vi "Check Sum Test_01.vi"(10 "Array":string[](array[string]), 11 "ToolString Input":string="$AGENT,53,VS-62U009+VS-69W014*71") -> (1 "ToolStringOut_01":string, 2 "ChkSum":string, 3 "x = y?":bool)   [LabVIEW 2019]
panel:
  out "ChkSum2":string
  out "ChkSum1":string
  out "ASCII 格式輸出 2":string
  out "ASCII 格式輸出":string
  out "number 3":u32
  out "number 2":u32
  out "Rad In Reg 2":string
  out "hex integer string":string[](array[string])
  out "unsigned byte array":u8[](array[numeric]) format="%x"
  out "Rad In Reg":string
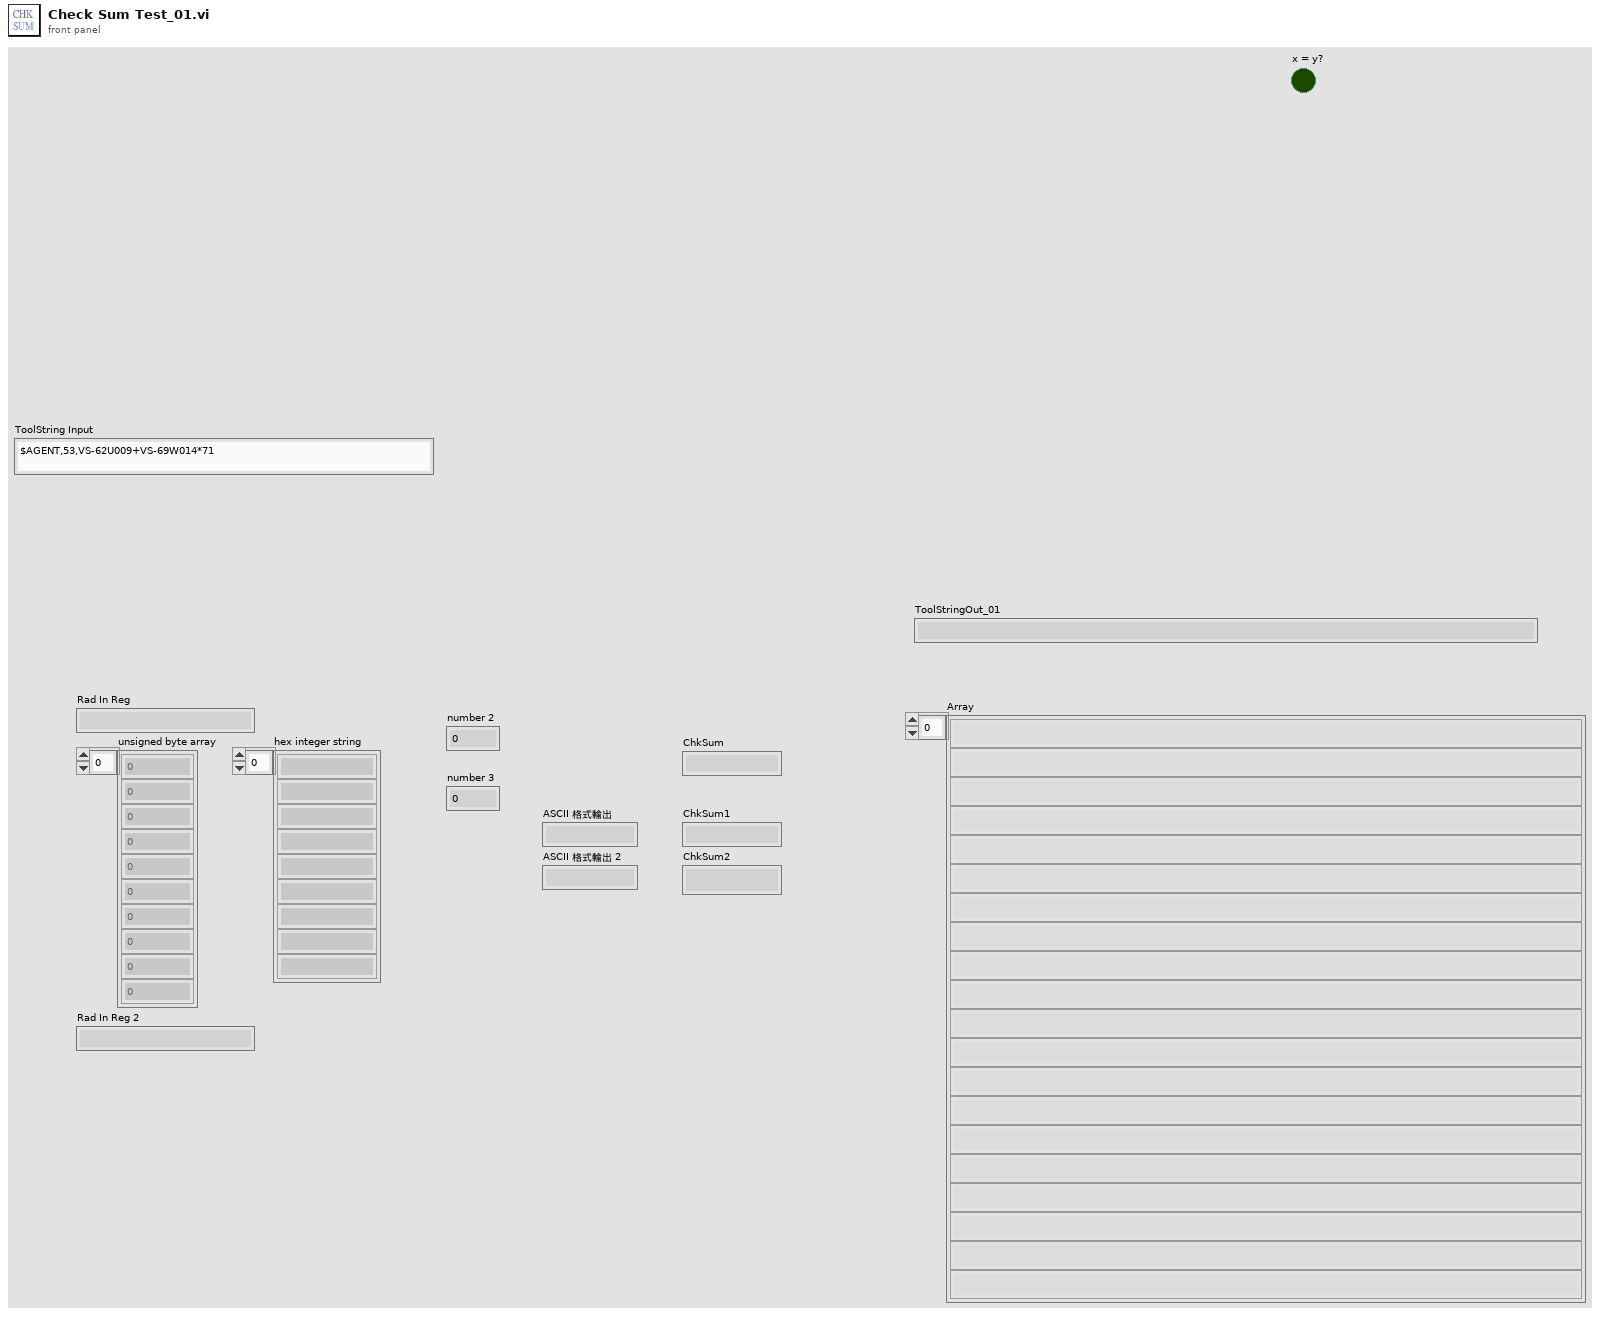
[diagram p1: front panel]
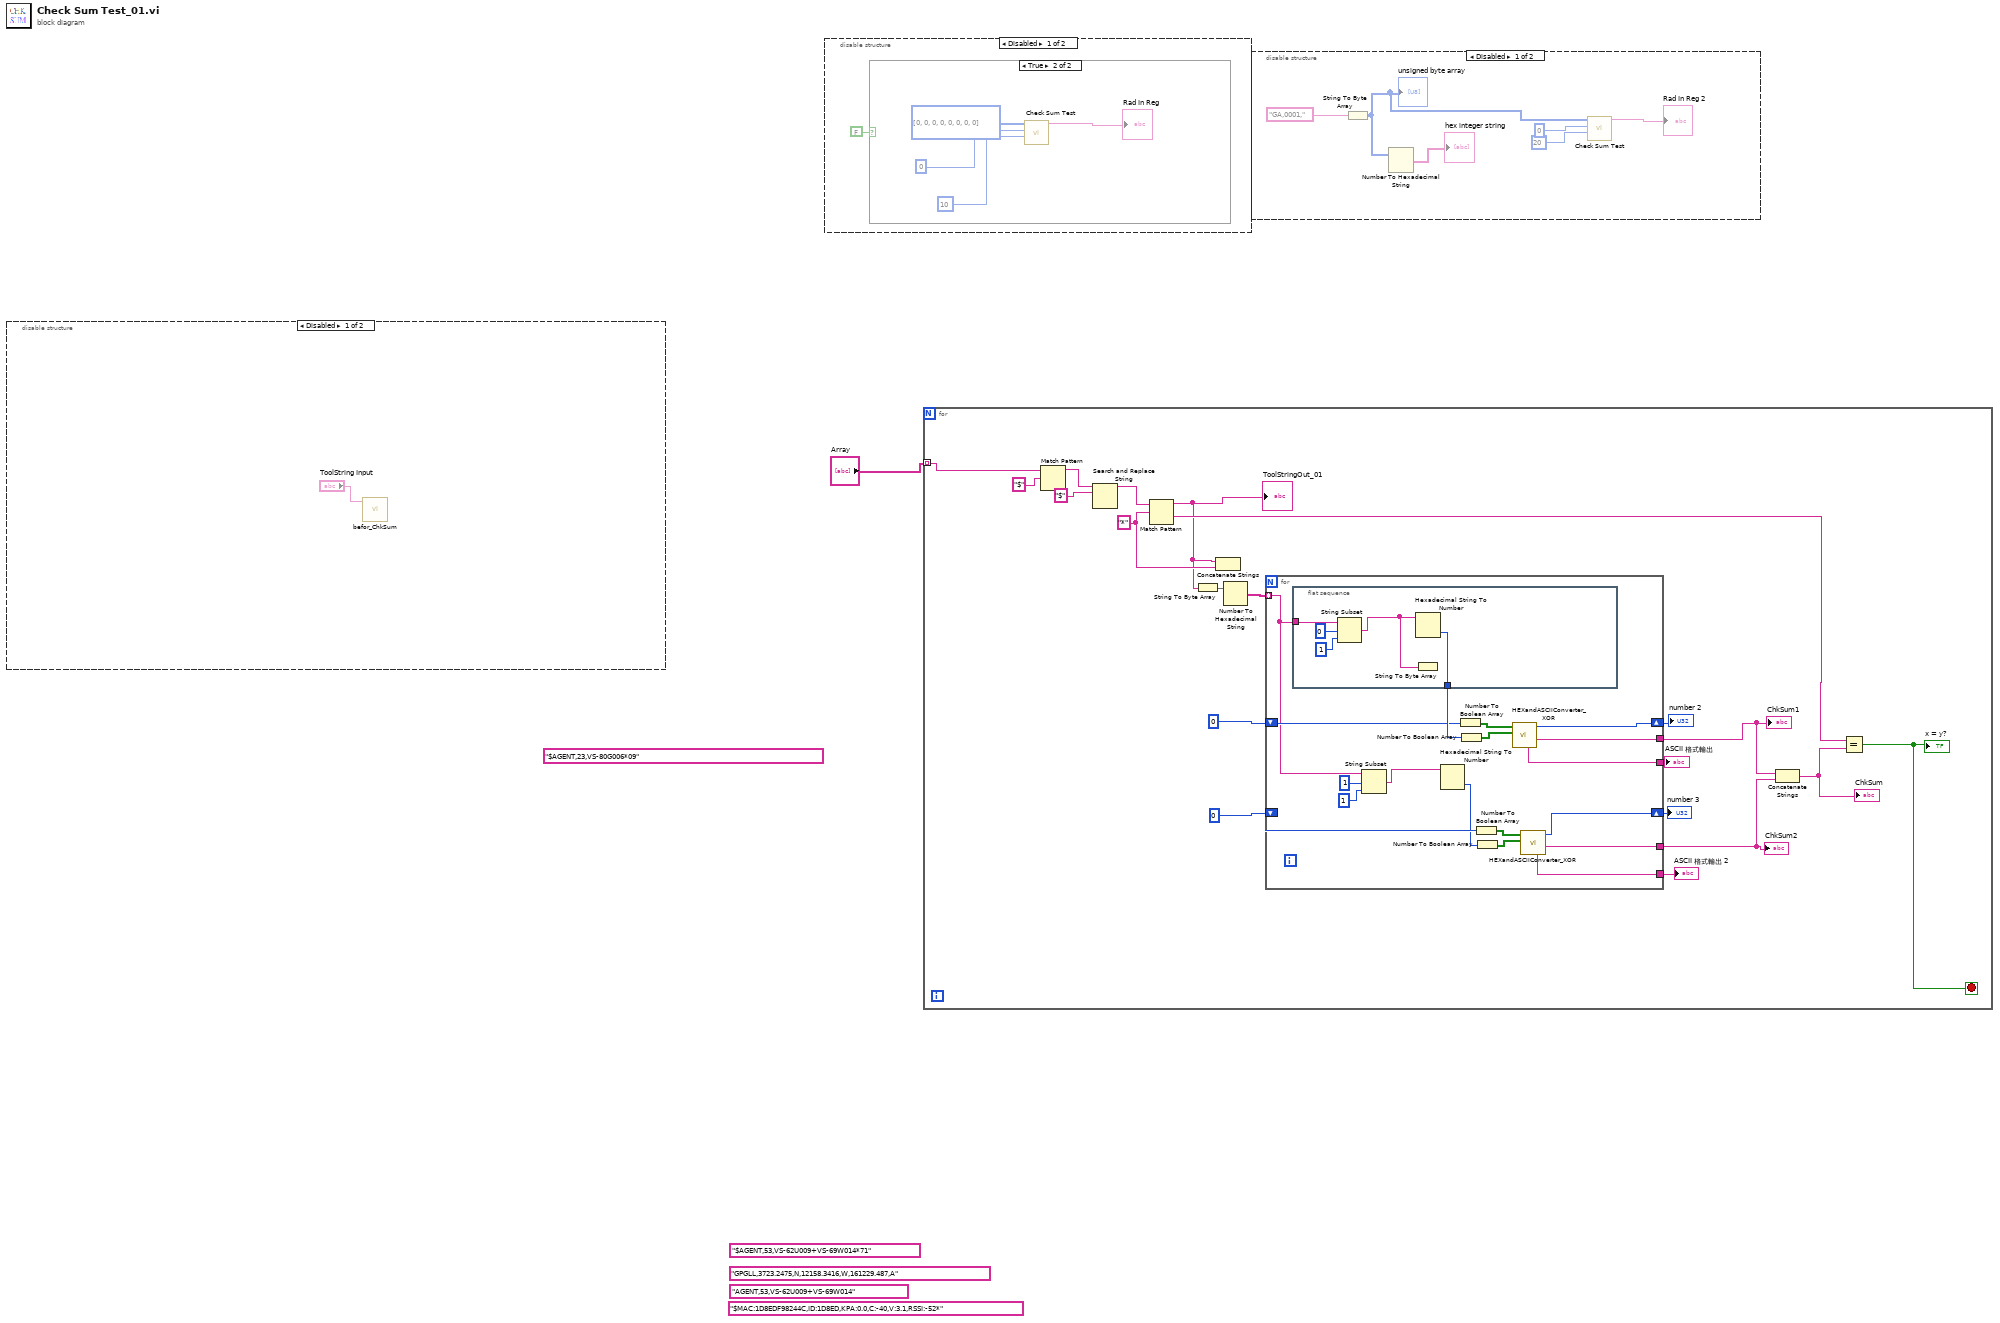
[diagram p0: block diagram]
diagram:
  (unwired) "$AGENT,23,VS-80G006*09"
  (unwired) "$AGENT,53,VS-62U009+VS-69W014*71"
  (unwired) "$MAC:1D8EDF98244C,ID:1D8ED,KPA:0.0,C:-40,V:3.1,RSSI:-52*"
  (unwired) "GPGLL,3723.2475,N,12158.3416,W,161229.487,A"
  (unwired) "AGENT,53,VS-62U009+VS-69W014"
  n1 = disable-structure shown="Disabled" {
    frame Disabled {
      n2 = call "befor_ChkSum.vi"("ToolString Input"="ToolString Input") -> ()  [unwired: 10 in, 1 out]
    }
    frame Enabled {
    }
  }
  n3 = disable-structure shown="Disabled" {
    frame Disabled {
      n4 = case shown="True" FALSE {
        frame False {
        }
        frame True {
          n5 = call "Check Sum Test.vi"("length"=10, "index"=0, "Input Registers Arr"=u16[] [0, 0, 0, 0, 0, 0, 0, 0]) -> ("Rad In Reg"=→"Rad In Reg":string)  [unwired: 8 in]
        }
      }
    }
    frame Enabled {
    }
  }
  n6 = for {
    tunnel: "Array" -> [w10] mode=indexing
    stop <- w9 stop-if-true
    w15 = "*" ("regular expression")
    n7 = Match Pattern(string=w10, regular expression="$") -> (before substring=w17:string)  [unwired: 1 in, 3 out]
    n8 = Search and Replace String(input string=w17, search string="$" ("regular expression")) -> (result string=w16:string)  [unwired: 6 in, 3 out]
    n9 = Match Pattern(string=w16, regular expression=w15) -> (before substring=w8:string, after substring=w12:string)  [unwired: 1 in, 2 out]
    "ToolStringOut_01" <- w8
    n10 = String To Byte Array(string=w8) -> (unsigned byte array=w23:u8[])
    n11 = Concatenate Strings(w8, w15) -> ()  [unwired: 1 out]
    n12 = Number To Hexadecimal String(2:w23) -> (0:w20:string[])  [unwired: 1 in]
    n13 = for {
      tunnel: w20 -> [w37] mode=indexing
      shift-right: [w41] -> w26
      shift-left: 0 -> [w42]
      shift-right: [w32] -> w24
      shift-left: 0 -> [w34]
      tunnel: [w31] -> w22
      tunnel: [w30] -> w21
      tunnel: [w29] -> w14
      tunnel: [w28] -> w13
      n14 = flat-sequence {
        tunnel: w37 -> [w48]
        tunnel: [w46] -> w43
        frame #0 {
          n15 = String Subset(string=w48, offset (0)=0, length (rest)=1) -> (substring=w47:string)
          n16 = Hexadecimal String To Number(string=w47) -> (number=w46:u32)  [unwired: 2 in, 1 out]
          n17 = String To Byte Array(string=w47) -> ()  [unwired: 1 out]
        }
      }
      n18 = String Subset(string=w37, offset (0)=1, length (rest)=1) -> (substring=w40:string)
      n19 = Hexadecimal String To Number(string=w40) -> (number=w33:u32)  [unwired: 2 in, 1 out]
      n20 = Number To Boolean Array(number=w42) -> (Boolean array=w45:bool[])
      n21 = Number To Boolean Array(number=w43) -> (Boolean array=w44:bool[])
      n22 = Number To Boolean Array(number=w34) -> (Boolean array=w35:bool[])
      n23 = Number To Boolean Array(number=w33) -> (Boolean array=w36:bool[])
      n24 = call "HEXandASCIIConverter_XOR.vi"("Boolean array2 in"=w44, "Boolean array1 in"=w45) -> ("hex integer string"=w29:string, "number"=w41:u32, "ASCII 格式輸出"=w31:string)  [unwired: 6 in, 1 out]
      n25 = call "HEXandASCIIConverter_XOR.vi"("Boolean array2 in"=w36, "Boolean array1 in"=w35) -> ("hex integer string"=w28:string, "number"=w32:u32, "ASCII 格式輸出"=w30:string)  [unwired: 6 in, 1 out]
    }
    "number 2" <- w26
    "number 3" <- w24
    "ASCII 格式輸出" <- w22
    "ASCII 格式輸出 2" <- w21
    "ChkSum1" <- w14
    "ChkSum2" <- w13
    n26 = Concatenate Strings(w14, w13) -> (w11:string)
    "ChkSum" <- w11
    n27 = Equal?(x=w12, y=w11) -> (x = y?=w9:bool)
    "x = y?" <- w9
  }
  n28 = disable-structure shown="Disabled" {
    frame Disabled {
      n29 = String To Byte Array(string="GA,0001,") -> (unsigned byte array=w54:u8[])
      "unsigned byte array" <- w54
      n30 = Number To Hexadecimal String(2:w54) -> (0:→"hex integer string":string[])  [unwired: 1 in]
      n31 = call "Check Sum Test.vi"("length"=20, "index"=0, "Input Registers Arr"=w54) -> ("Rad In Reg"=→"Rad In Reg 2":string)  [unwired: 8 in]
    }
    frame Enabled {
    }
  }
